vi "Passaggio decimali in binario.vi"(1 "Numero 2":dbl, 2 "Numero 1":dbl) -> (0 "num1+num2\nin binario":i8 format="%b")   [LabVIEW 2012]
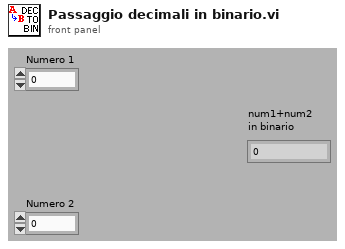
[diagram p1: front panel]
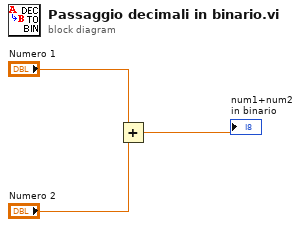
[diagram p0: block diagram]
diagram:
  n1 = Add(x="Numero 1", y="Numero 2") -> (x+y=→"num1+num2\nin binario":dbl)
